vi "FTW-ProjectItem-Tag-Delete.vi"(0 "ProjectItem":refnum<vi>, 5 "Tag Name Regex Matches to Delete":string, 11 "error in":errorcluster) -> (4 "ProjectItem out":refnum<vi>, 6 "Tags Deleted":string[](array[string]), 15 "error out":errorcluster)   [LabVIEW 2012]
panel:
  # "Inputs"
  # "Outputs"
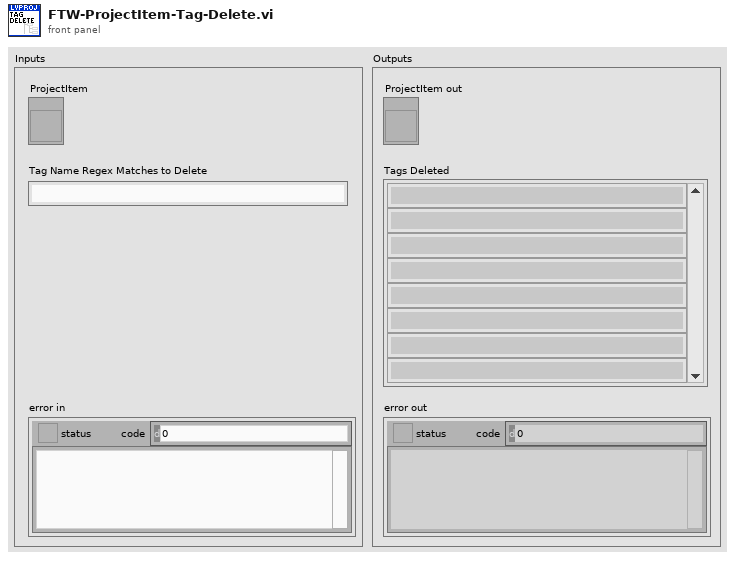
[diagram p1: front panel]
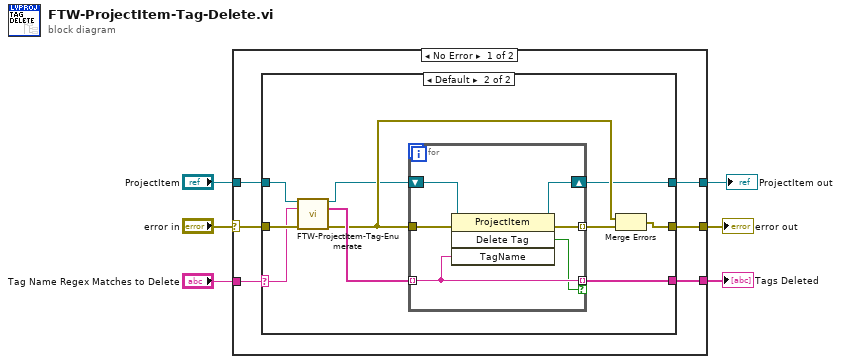
[diagram p0: block diagram]
diagram:
  n1 = case shown="No Error" "error in" {
    selector: "error in" -> [w12 w32]
    tunnel: [w11 w32] -> w6
    tunnel: "Tag Name Regex Matches to Delete" -> [w10 _]
    tunnel: [w9 _] -> w3
    tunnel: "ProjectItem" -> [w8 w31]
    tunnel: [w7 w31] -> w1
    frame No Error {
      n2 = case shown="Default" w10 {
        selector: w10 -> [_ w22]
        tunnel: w8 -> [w13 w19]
        tunnel: w12 -> [w14 w23]
        tunnel: [w14 w18] -> w11
        tunnel: [_ w20] -> w9
        tunnel: [w13 w16] -> w7
        frame "" {
        }
        frame Default {
          n3 = call "FTW-ProjectItem-Tag-Enumerate.vi"("ProjectItem"=w19, "Tag Name Regex Filter (blank returns all tags)"=w22, "error in"=w23) -> ("ProjectItem out"=w15:refnum<vi>, "Matching Tags"=w21:string[], "error out"=w17:errorcluster)  [unwired: 9 in, 1 out]
          n4 = for {
            tunnel: w21 -> [w27] mode=indexing
            tunnel: [w27] -> w20 mode=indexing if=w26
            tunnel: w17 -> [w28]
            tunnel: [w29] -> w24 mode=indexing
            shift-right: [w25] -> w16
            shift-left: w15 -> [w30]
            n5 = invoke class="ProjectItem" method="Delete Tag"(reference=w30, error in=w28, "TagName"=w27) -> (reference out=w25:refnum<vi>, error out=w29:errorcluster, "DeleteTag"=w26:bool)  [unwired: 1 in, 1 out]
          }
          n6 = Merge Errors(w17, w24) -> (w18:errorcluster)
        }
      }
    }
    frame Error {
    }
  }
  "error out" <- w6
  "Tags Deleted" <- w3
  "ProjectItem out" <- w1
